vi "Get_User_Filename_and_Path.vi"(8 "error in (no error)":errorcluster) -> (0 "error out":errorcluster, 2 "TXT File Path":path, 3 "CSV File Path":path)   [LabVIEW 2021]
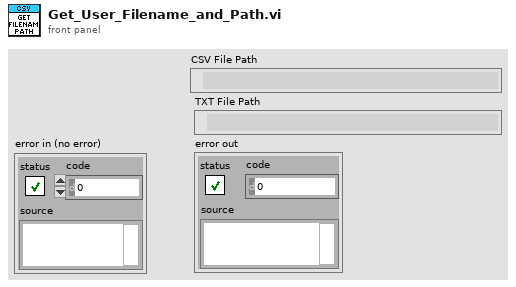
[diagram p1: front panel]
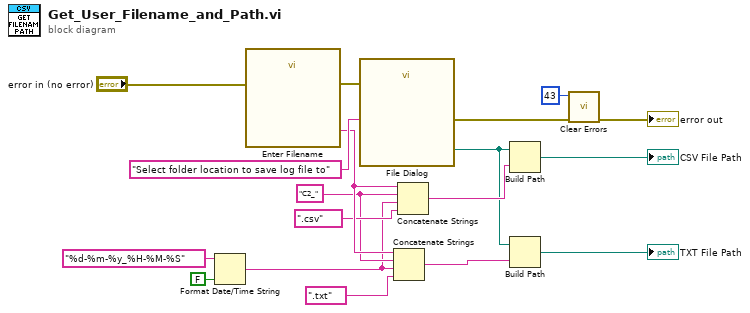
[diagram p0: block diagram]
diagram:
  w2 = "C2_" ("string")
  n1 = Format Date/Time String(time format string (%c)="%d-%m-%y_%H-%M-%S", UTC format=FALSE) -> (date/time string=w1:string)  [unwired: 1 in]
  n2 = call "Enter Filename"("error in (no error)"="error in (no error)") -> ("Filename"=w11:string, "error out"=w18:errorcluster)  [unwired: 16 in, 1 out]
  n3 = call "File Dialog"("prompt"="Select folder location to save log file to", "error in"=w18) -> ("selected path"=w12:path, "error out"=w9:errorcluster)  [unwired: 10 in, 2 out]
  n4 = Concatenate Strings(w11, w2, w1, ".txt" ("string")) -> (w13:string)
  n5 = Concatenate Strings(w11, w2, w1, ".csv" ("string")) -> (w16:string)
  n6 = Build Path(base path=w12, name or relative path=w16) -> (appended path=→"CSV File Path":path)
  n7 = Build Path(base path=w12, name or relative path=w13) -> (appended path=→"TXT File Path":path)
  n8 = call <vilib>:"Clear Errors.vi"("error in (no error)"=w9, "specific error code to clear (0: all)"=43) -> ("error out"=→"error out":errorcluster)  [unwired: 4 in, 1 out]
